vi "Get Waveform Data from Reference.vi"(5 "Waveform Data Reference":refnum<data-value>, 9 "error in (no error)":errorcluster) -> (6 "Waveform Data":cluster{"t0":dbl, "dt":dbl, "y":csg[]}, 10 "error out":errorcluster)   [LabVIEW 2019, in "Common.lvlib"]
doc: "Retrieves the <b>Waveform Data</b> from <b>Waveform Data Reference</b>."
uses:
  Common.lvlib
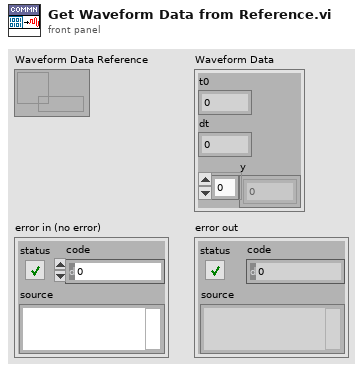
[diagram p1: front panel]
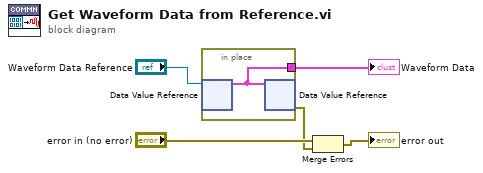
[diagram p0: block diagram]
diagram:
  n1 = in-place {
    in-place-border: [w6] -> w1
    n2 = in-place-dvr #1("Waveform Data Reference") -> (w6:cluster{"t0":dbl, "dt":dbl, "y":csg[]})  [unwired: 1 out]
    n3 = in-place-dvr #1(w6) -> (w2:errorcluster)  [unwired: 1 out]
  }
  "Waveform Data" <- w1
  n4 = Merge Errors("error in (no error)", w2) -> (→"error out":errorcluster)
